vi "getIndex.vi"(8 "error in (no error)":errorcluster, 9 "value":string, 10 "key":string, 11 "VElement":variant) -> (0 "error out":errorcluster, 3 "indexOut":i32)   [LabVIEW 2015, in "Zen Analytics.lvclass"]
uses:
  Zen Analytics.lvclass
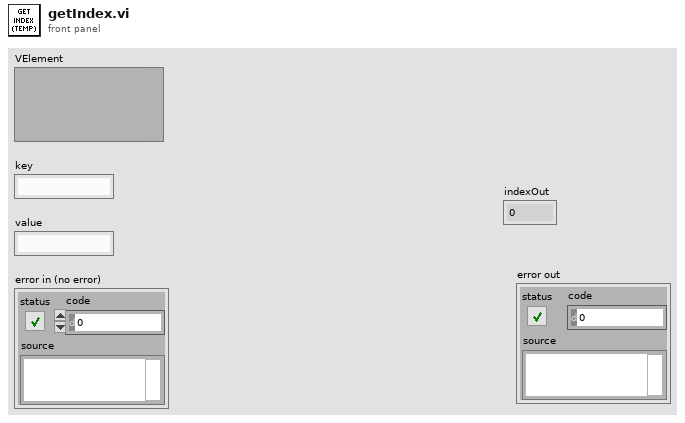
[diagram p1: front panel]
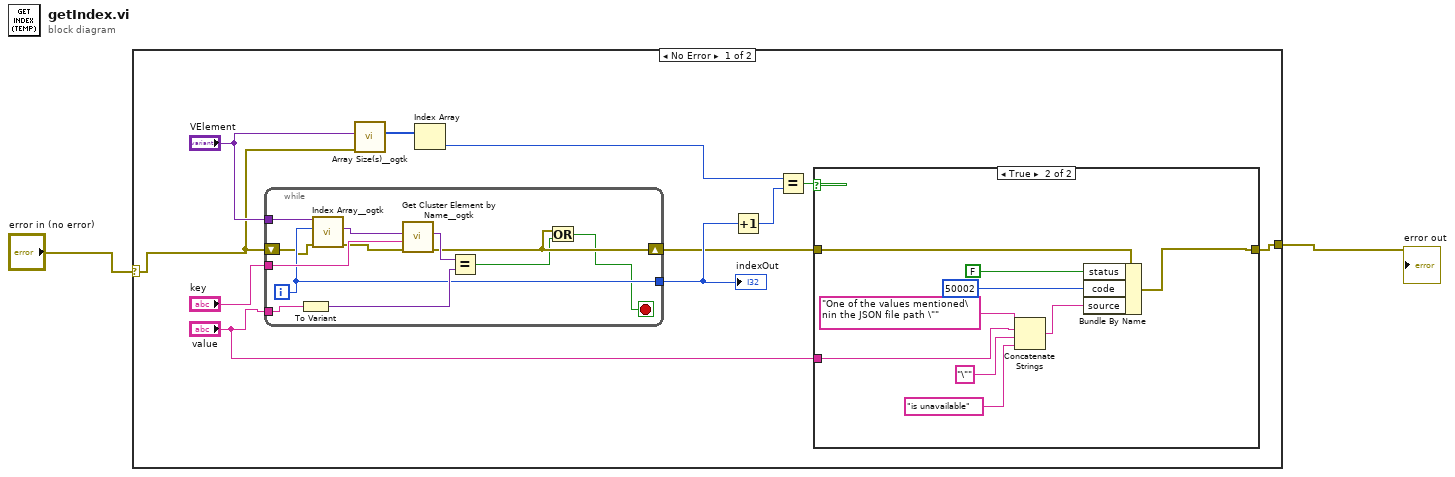
[diagram p0: block diagram]
diagram:
  n1 = case shown="No Error" "error in (no error)" {
    selector: "error in (no error)" -> [w11 w36]
    tunnel: [w3 w36] -> w1
    frame No Error {
      n2 = while {
        tunnel: "VElement" -> [w35]
        tunnel: "key" -> [w33]
        tunnel: "value" -> [w32]
        tunnel: [w29] -> w10
        shift-right: [w28] -> w6
        shift-left: w11 -> [w25]
        i -> [w29]
        stop <- w26 stop-if-true
        n3 = To Variant(anything=w32) -> (Variant=w30:variant)
        n4 = call <userlib>:"Index Array__ogtk.vi"("error in (no error)"=w25, "Index (1D)"=w29, "MultiD Array"=w35) -> ("error out"=w24:errorcluster, "Array Element"=w34:variant)  [unwired: 7 in]
        n5 = call <userlib>:"Get Cluster Element by Name__ogtk.vi"("error in (no error)"=w24, "Element Name"=w33, "Cluster"=w34) -> ("error out"=w28:errorcluster, "VElement"=w31:variant)  [unwired: 6 in, 1 out]
        n6 = Equal?(x=w31, y=w30) -> (x = y?=w27:bool)
        n7 = Or(x=w28, y=w27) -> (x .or. y?=w26:bool)
      }
      "indexOut" <- w10
      n8 = call <userlib>:"Array Size(s)__ogtk.vi"("error in (no error)"=w11, "Array"="VElement") -> ("Size(s)"=w12:u32[])  [unwired: 7 in, 2 out]
      n9 = Index Array(array=w12) -> (element=w8:u32)  [unwired: 1 in]
      n10 = Increment(x=w10) -> (x+1=w9:i32)
      n11 = Equal?(x=w8, y=w9) -> (x = y?=w7:bool)
      n12 = case shown="True" w7 {
        tunnel: w6 -> [w14 w23]
        tunnel: "value" -> [_ w19]
        tunnel: [w14 w15] -> w3
        frame False {
        }
        frame True {
          n13 = Concatenate Strings("One of the values mentioned\nin the JSON file path \"" ("source"), w19, "\"" ("string"), "is unavailable" ("string")) -> (w18:string)
          n14 = Bundle By Name(cluster=w23, "status"=FALSE, "code"=50002, "source"=w18) -> (w15:errorcluster)
        }
      }
    }
    frame Error {
    }
  }
  "error out" <- w1
